vi "get_std_observing_modes.vi"(4 "error in (no error)":errorcluster, 6 "mode name":string, 7 "configuration file path":path) -> (0 "error out":errorcluster, 2 "Standard Mode Info":T1 {"grating angle" format="%.2f"})   [LabVIEW 2015]
uses:
  <vilib>/Utility/config.llb/Read Key (String).vi
  <vilib>/Utility/config.llb/Read Key (Double).vi
  <vilib>/Utility/config.llb/NI_LVConfig.lvlib
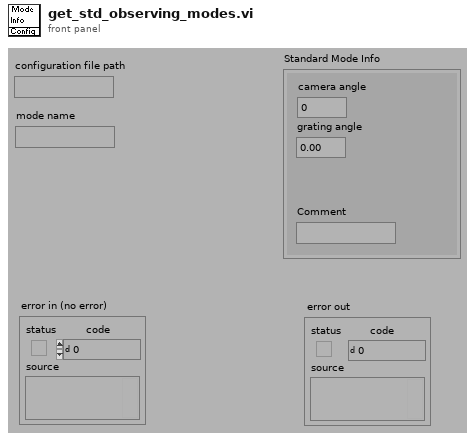
[diagram p1: front panel]
types:
  T1 = cluster{"Comment":string, "camera angle":dbl, "grating angle":dbl}
  T2 = typedef "NI_LVConfig.lvlib/Config Data RefNum.ctl" = refnum<k1>
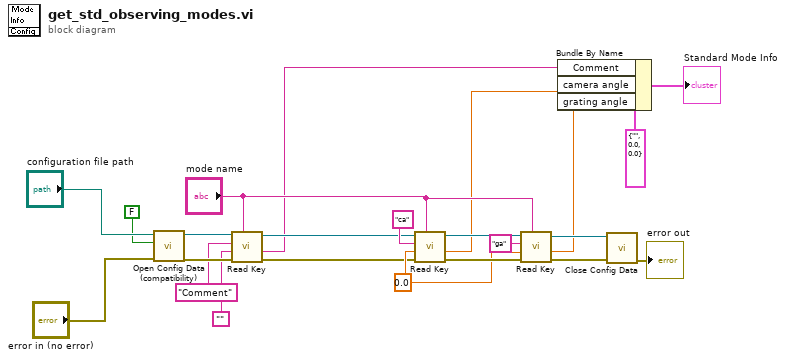
[diagram p0: block diagram]
diagram:
  w10 = 0.0
  n1 = call <vilib>:"Open Config Data (compatibility).vi"("error in (no error)"="error in (no error)", "create file if necessary (T)"=FALSE, "configuration file path"="configuration file path") -> ("error out"=w23:errorcluster, "refnum"=w22:T2)  [unwired: 6 in, 1 out]
  n2 = call-poly <vilib>:"Read Key.vi"("section"="mode name", "error in (no error)"=w23, "default value"="", "key"="Comment", "refnum"=w22) -> ("error out"=w6:errorcluster, "value"=w5:string, "refnum out"=w7:T2)  [unwired: 3 in, 1 out]
  n3 = call-poly <vilib>:"Read Key.vi"("section"="mode name", "error in (no error)"=w6, "default value"=w10, "key"="ca", "refnum"=w7) -> ("error out"=w13:errorcluster, "value"=w4:dbl, "refnum out"=w14:T2)  [unwired: 3 in, 1 out]
  n4 = call-poly <vilib>:"Read Key.vi"("section"="mode name", "error in (no error)"=w13, "default value"=w10, "key"="ga", "refnum"=w14) -> ("error out"=w9:errorcluster, "value"=w3:dbl, "refnum out"=w8:T2)  [unwired: 3 in, 1 out]
  n5 = Bundle By Name(cluster=T1 {"Comment"="", "camera angle"=0.0, "grating angle"=0.0} ("Standard Mode Info"), "Comment"=w5, "camera angle"=w4, "grating angle"=w3) -> (→"Standard Mode Info":T1)
  n6 = call <vilib>:"Close Config Data.vi"("error in (no error)"=w9, "refnum"=w8) -> ("error out"=→"error out":errorcluster)  [unwired: 8 in, 1 out]
